vi "session_error.vi"() -> ()   [LabVIEW 2017]
doc: "Illustrates how errors can be written to and read from libssh2."
uses:
  libssh2/libssh2_init_default.vi
  libssh2/libssh2_session_init_ex.vi
  libssh2/libssh2.lvlib
panel:
  in  "error message":string="Error!"
  in  "error code":i32=-1
  out "last error message":string
  out "last error code":i32
  out "error out":errorcluster
  # "Set the initial error state for the next function call."
  # "Get the last error state."
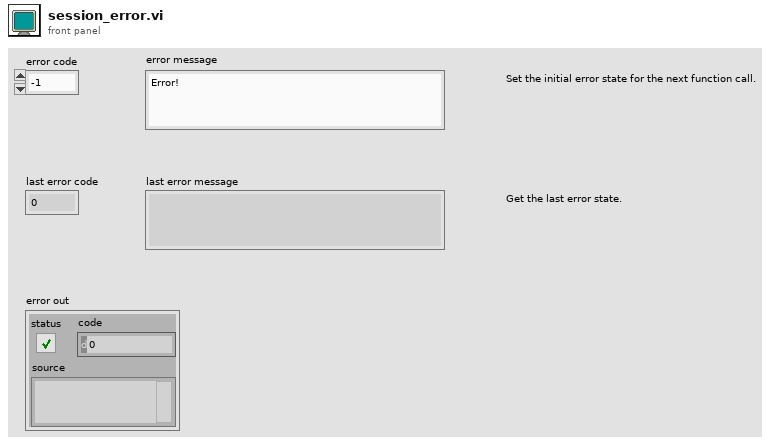
[diagram p1: front panel]
types:
  T1 = typedef "libssh2.lvlib/Session Refnum.ctl" = refnum<k1>
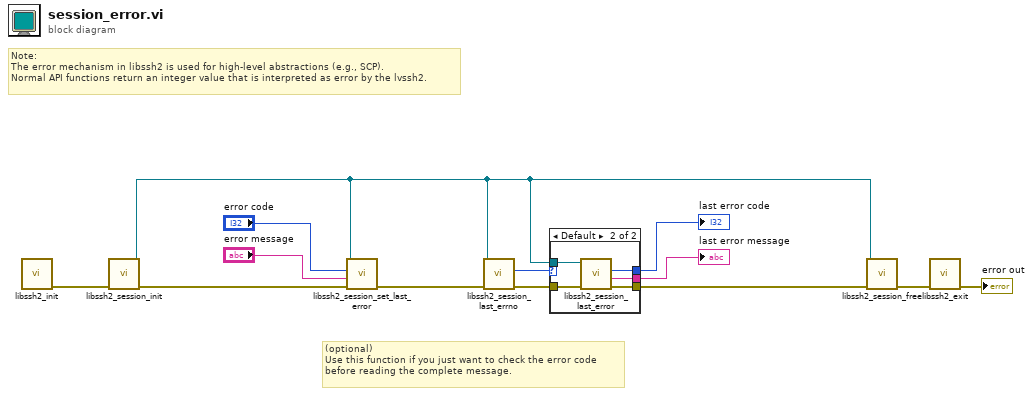
[diagram p0: block diagram]
diagram:
  # "(optional)\nUse this function if you just want to check the error code\nbefore reading the complete message."
  # "Note:\nThe error mechanism in libssh2 is used for high-level abstractions (e.g., SCP).\nNormal API functions return an integer value that is interpreted as error by the lvssh2."
  n1 = call-poly "libssh2_init.vi"() -> ("error out"=w13:errorcluster)  [unwired: 11 in]
  n2 = call "libssh2_session_init.vi"("error in (no error)"=w13) -> ("error out"=w11:errorcluster, "session"=w8:T1)  [unwired: 9 in]
  n3 = call "libssh2_session_set_last_error.vi"("error in (no error)"=w11, "error message"="error message", "error code"="error code", "session"=w8) -> ("error out"=w4:errorcluster)  [unwired: 7 in]
  n4 = call "libssh2_session_last_errno.vi"("error in (no error)"=w4, "session"=w8) -> ("error out"=w5:errorcluster, "error code"=w2:i32)  [unwired: 8 in]
  n5 = case shown="Default" w2 {
    tunnel: [_ w19] -> w10
    tunnel: [_ w18] -> w9
    tunnel: w8 -> [_ w17]
    tunnel: w5 -> [w14 w16]
    tunnel: [w14 w15] -> w3
    frame 0 {
    }
    frame Default {
      n6 = call "libssh2_session_last_error.vi"("error in (no error)"=w16, "session"=w17) -> ("error out"=w15:errorcluster, "error message"=w18:string, "error code"=w19:i32)  [unwired: 7 in]
    }
  }
  "last error code" <- w10
  "last error message" <- w9
  n7 = call "libssh2_session_free.vi"("error in (no error)"=w3, "session"=w8) -> ("error out"=w12:errorcluster)  [unwired: 9 in]
  n8 = call "libssh2_exit.vi"("error in (no error)"=w12) -> ("error out"=→"error out":errorcluster)  [unwired: 10 in]
